vi "Notifier-with-memory-camera.vi"(8 "error in":errorcluster, 10 "Timeout [ms]":i32, 11 "Notifier in":refnum<notifier>) -> (0 "error IO":errorcluster, 2 "Notification":T1)   [LabVIEW 2013, in "CameraVision.lvlib" / "CV-UI.lvclass"]
doc: "Polymorphic type of Notifier-with-memory vi.\n\nAccepts a notifier reference for an instance of the type-defined control 'Camera selector'.\nThe vi listens for 'Timeout' miliseconds for a new message on the notifier.\nIf no message arrives or arrived before calling the vi, the last received message is returned.\n\nThe default message is 'Camera 1'."
uses:
  CV-UI.lvclass
  Camera-selector.ctl
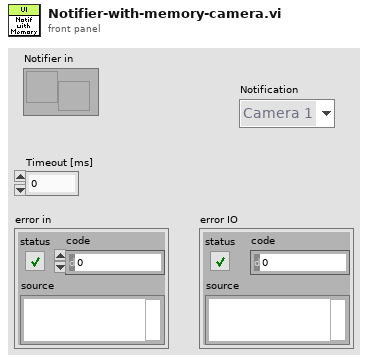
[diagram p1: front panel]
types:
  T1 = typedef "CameraVision.lvlib/CV-UI.lvclass/Camera-selector.ctl" = enum16{"Camera 1", "Camera 2"}
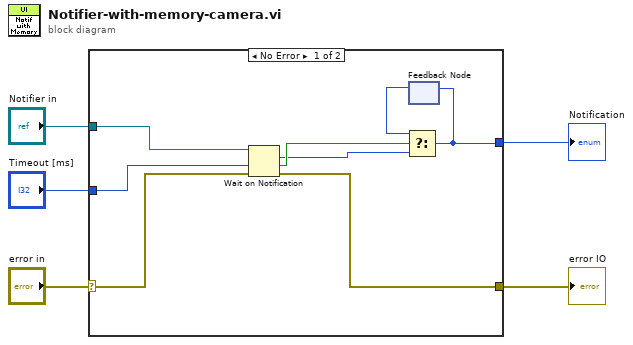
[diagram p0: block diagram]
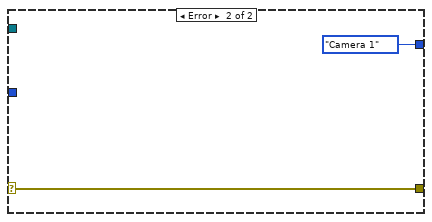
[diagram p2: hidden frame]
diagram:
  n1 = case shown="No Error" "error in" {
    selector: "error in" -> [w6 w15]
    tunnel: [w13 w15] -> w5
    tunnel: "Timeout [ms]" -> [w12 _]
    tunnel: "Notifier in" -> [w8 _]
    tunnel: [w7 Camera-selector."Camera 1" ("Camera selector")] -> w2
    frame No Error {
      n2 = Wait on Notification(notifier=w8, timeout in ms (-1)=w12, error in (no error)=w6) -> (notification=w10:T1, timed out?=w11:bool, error out=w13:errorcluster)  [unwired: 1 in, 1 out]
      n3 = feedback #1() -> (w9:T1)  [unwired: 1 in]
      n4 = Select(t=w9, s=w11, f=w10) -> (s? t:f=w7:T1)
      n5 = feedback-in #1(w7) -> ()
    }
    frame Error {
    }
  }
  "error IO" <- w5
  "Notification" <- w2
